vi "计算结果到报表.vi"(3 "计算参数":T1, 4 "试验模式":string, 5 "试验报表路径":path) -> ()   [LabVIEW 2013]
doc: "该函数将计算所得的参数写入到试验报表的文本文档里。"
uses:
  <vilib>/Utility/config.llb/Write Key (Double).vi
  <vilib>/Utility/config.llb/NI_LVConfig.lvlib
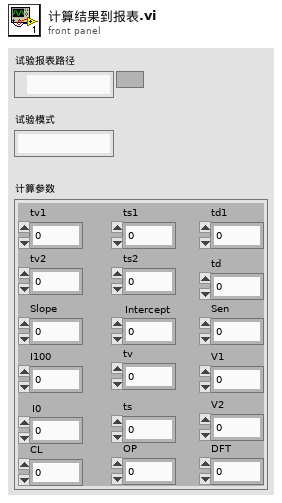
[diagram p1: front panel]
types:
  T1 = cluster{"tv1":dbl, "tv2":dbl, "tv":dbl, "ts1":dbl, "ts2":dbl, "ts":dbl, "td1":dbl, "td":dbl, "Slope":dbl, "Intercept":dbl, "I100":dbl, "I0":dbl, "Sen":dbl, "V1":dbl, "V2":dbl, "CL":dbl, "OP":dbl, "DFT":dbl}
  T2 = typedef "NI_LVConfig.lvlib/Config Data RefNum.ctl" = refnum<k1>
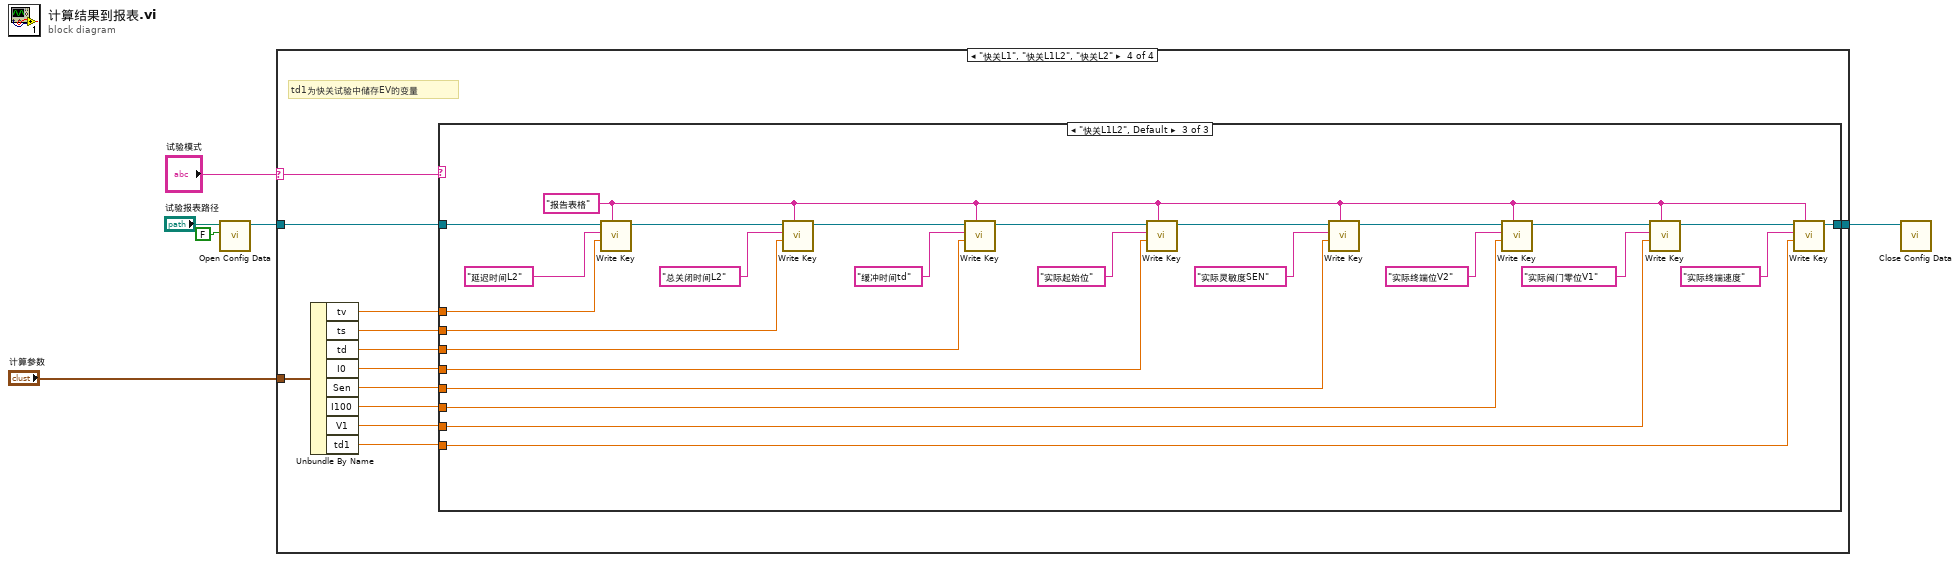
[diagram p0: block diagram]
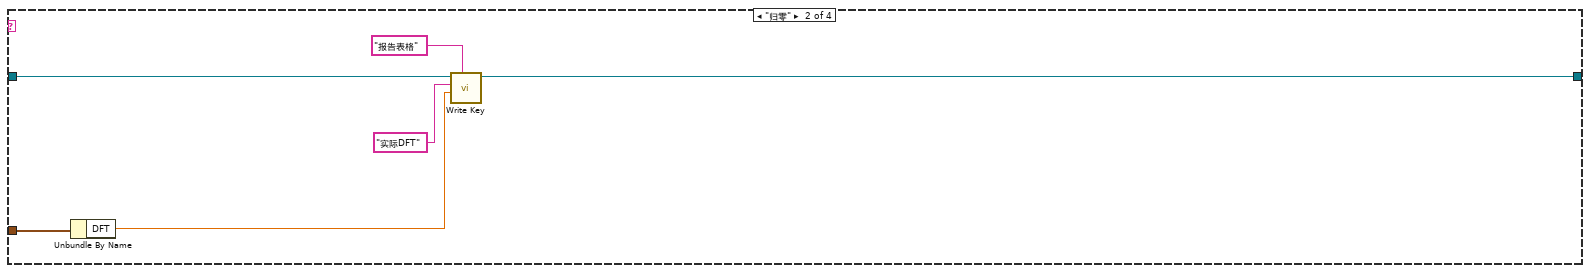
[diagram p3: hidden frame]
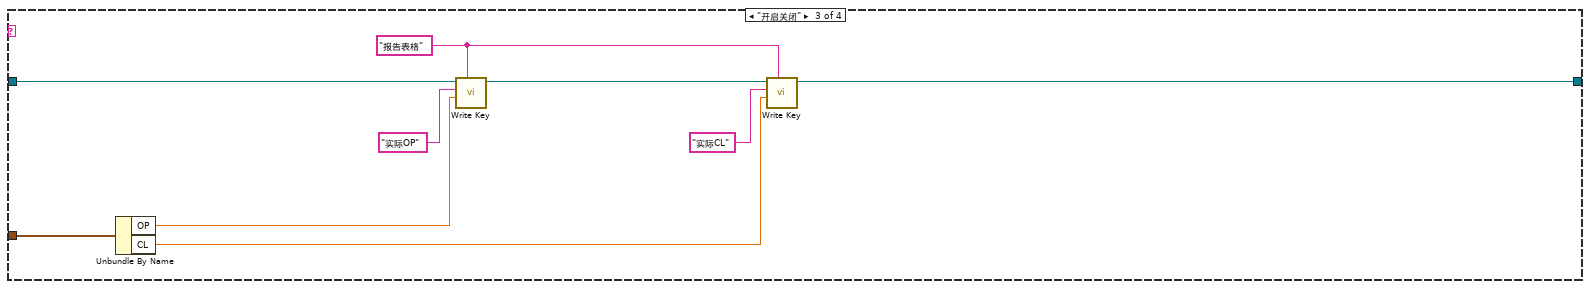
[diagram p4: hidden frame]
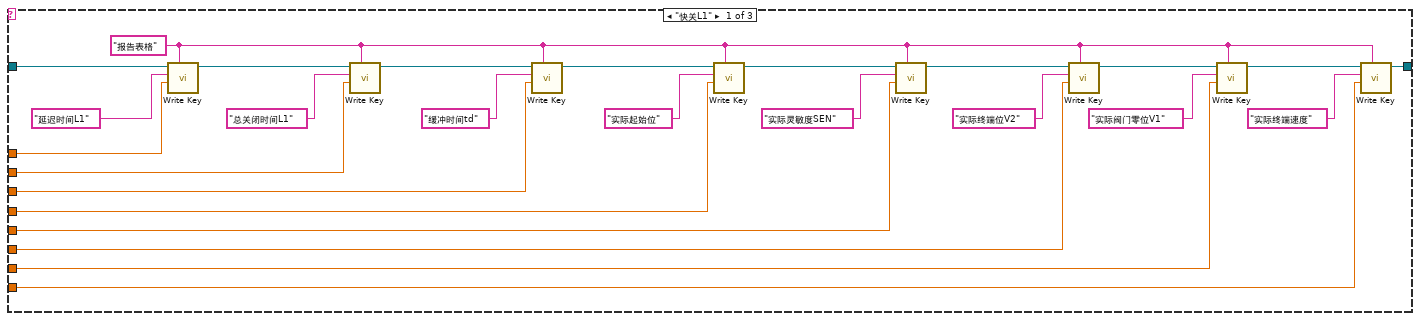
[diagram p5: hidden frame]
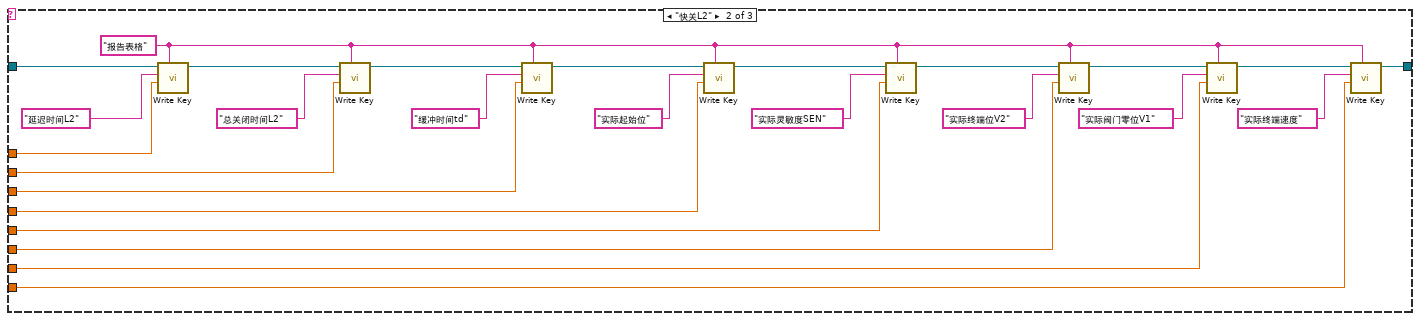
[diagram p6: hidden frame]
diagram:
  n1 = call <vilib>:"Open Config Data.vi"("create file if necessary (T)"=FALSE, "configuration file path"="试验报表路径") -> ("refnum"=w3:T2)  [unwired: 7 in, 2 out]
  n2 = case shown="\"快关L1\", \"快关L1L2\", \"快关L2\"" "试验模式" {
    selector: "试验模式" -> [_ _ _ w34]
    tunnel: "计算参数" -> [_ w13 w22 w33]
    tunnel: w3 -> [w7 w10 w15 w32]
    tunnel: [w7 w9 w14 w31] -> w2
    frame "步响应", Default {
    }
    frame "归零" {
      n3 = Unbundle By Name(w13) -> ("DFT"=w8:dbl)
      n4 = call-poly <vilib>:"Write Key.vi"("section"="报告表格", "value"=w8, "key"="实际DFT", "refnum"=w10) -> ("refnum out"=w9:T2)  [unwired: 5 in, 2 out]
    }
    frame "开启关闭" {
      w19 = "报告表格"
      n5 = Unbundle By Name(w22) -> ("OP"=w17:dbl, "CL"=w16:dbl)
      n6 = call-poly <vilib>:"Write Key.vi"("section"=w19, "value"=w17, "key"="实际OP", "refnum"=w15) -> ("refnum out"=w18:T2)  [unwired: 5 in, 2 out]
      n7 = call-poly <vilib>:"Write Key.vi"("section"=w19, "value"=w16, "key"="实际CL", "refnum"=w18) -> ("refnum out"=w14:T2)  [unwired: 5 in, 2 out]
    }
    frame "快关L1", "快关L1L2", "快关L2" {
      # "td1为快关试验中储存EV的变量"
      n8 = Unbundle By Name(w33) -> ("tv"=w30:dbl, "ts"=w29:dbl, "td"=w28:dbl, "I0"=w23:dbl, "Sen"=w24:dbl, "I100"=w25:dbl, "V1"=w26:dbl, "td1"=w27:dbl)
      n9 = case shown="\"快关L1L2\", Default" w34 {
        tunnel: w32 -> [w44 w86 w88]
        tunnel: [w43 w69 w87] -> w31
        tunnel: w30 -> [w35 w84 w89]
        tunnel: w29 -> [w36 w76 w90]
        tunnel: w28 -> [w37 w75 w91]
        tunnel: w23 -> [w38 w74 w92]
        tunnel: w24 -> [w39 w73 w93]
        tunnel: w25 -> [w40 w72 w94]
        tunnel: w26 -> [w41 w71 w95]
        tunnel: w27 -> [w42 w70 w96]
        frame "快关L1" {
          w45 = "报告表格"
          n10 = call-poly <vilib>:"Write Key.vi"("section"=w45, "value"=w35, "key"="延迟时间L1", "refnum"=w44) -> ("refnum out"=w52:T2)  [unwired: 5 in, 2 out]
          n11 = call-poly <vilib>:"Write Key.vi"("section"=w45, "value"=w36, "key"="总关闭时间L1", "refnum"=w52) -> ("refnum out"=w51:T2)  [unwired: 5 in, 2 out]
          n12 = call-poly <vilib>:"Write Key.vi"("section"=w45, "value"=w37, "key"="缓冲时间td", "refnum"=w51) -> ("refnum out"=w50:T2)  [unwired: 5 in, 2 out]
          n13 = call-poly <vilib>:"Write Key.vi"("section"=w45, "value"=w38, "key"="实际起始位", "refnum"=w50) -> ("refnum out"=w49:T2)  [unwired: 5 in, 2 out]
          n14 = call-poly <vilib>:"Write Key.vi"("section"=w45, "value"=w39, "key"="实际灵敏度SEN", "refnum"=w49) -> ("refnum out"=w48:T2)  [unwired: 5 in, 2 out]
          n15 = call-poly <vilib>:"Write Key.vi"("section"=w45, "value"=w40, "key"="实际终端位V2", "refnum"=w48) -> ("refnum out"=w47:T2)  [unwired: 5 in, 2 out]
          n16 = call-poly <vilib>:"Write Key.vi"("section"=w45, "value"=w41, "key"="实际阀门零位V1", "refnum"=w47) -> ("refnum out"=w46:T2)  [unwired: 5 in, 2 out]
          n17 = call-poly <vilib>:"Write Key.vi"("section"=w45, "value"=w42, "key"="实际终端速度", "refnum"=w46) -> ("refnum out"=w43:T2)  [unwired: 5 in, 2 out]
        }
        frame "快关L2" {
          w61 = "报告表格"
          n18 = call-poly <vilib>:"Write Key.vi"("section"=w61, "value"=w84, "key"="延迟时间L2", "refnum"=w86) -> ("refnum out"=w68:T2)  [unwired: 5 in, 2 out]
          n19 = call-poly <vilib>:"Write Key.vi"("section"=w61, "value"=w76, "key"="总关闭时间L2", "refnum"=w68) -> ("refnum out"=w67:T2)  [unwired: 5 in, 2 out]
          n20 = call-poly <vilib>:"Write Key.vi"("section"=w61, "value"=w75, "key"="缓冲时间td", "refnum"=w67) -> ("refnum out"=w66:T2)  [unwired: 5 in, 2 out]
          n21 = call-poly <vilib>:"Write Key.vi"("section"=w61, "value"=w74, "key"="实际起始位", "refnum"=w66) -> ("refnum out"=w65:T2)  [unwired: 5 in, 2 out]
          n22 = call-poly <vilib>:"Write Key.vi"("section"=w61, "value"=w73, "key"="实际灵敏度SEN", "refnum"=w65) -> ("refnum out"=w64:T2)  [unwired: 5 in, 2 out]
          n23 = call-poly <vilib>:"Write Key.vi"("section"=w61, "value"=w72, "key"="实际终端位V2", "refnum"=w64) -> ("refnum out"=w63:T2)  [unwired: 5 in, 2 out]
          n24 = call-poly <vilib>:"Write Key.vi"("section"=w61, "value"=w71, "key"="实际阀门零位V1", "refnum"=w63) -> ("refnum out"=w62:T2)  [unwired: 5 in, 2 out]
          n25 = call-poly <vilib>:"Write Key.vi"("section"=w61, "value"=w70, "key"="实际终端速度", "refnum"=w62) -> ("refnum out"=w69:T2)  [unwired: 5 in, 2 out]
        }
        frame "快关L1L2", Default {
          w97 = "报告表格"
          n26 = call-poly <vilib>:"Write Key.vi"("section"=w97, "value"=w89, "key"="延迟时间L2", "refnum"=w88) -> ("refnum out"=w104:T2)  [unwired: 5 in, 2 out]
          n27 = call-poly <vilib>:"Write Key.vi"("section"=w97, "value"=w90, "key"="总关闭时间L2", "refnum"=w104) -> ("refnum out"=w103:T2)  [unwired: 5 in, 2 out]
          n28 = call-poly <vilib>:"Write Key.vi"("section"=w97, "value"=w91, "key"="缓冲时间td", "refnum"=w103) -> ("refnum out"=w102:T2)  [unwired: 5 in, 2 out]
          n29 = call-poly <vilib>:"Write Key.vi"("section"=w97, "value"=w92, "key"="实际起始位", "refnum"=w102) -> ("refnum out"=w101:T2)  [unwired: 5 in, 2 out]
          n30 = call-poly <vilib>:"Write Key.vi"("section"=w97, "value"=w93, "key"="实际灵敏度SEN", "refnum"=w101) -> ("refnum out"=w100:T2)  [unwired: 5 in, 2 out]
          n31 = call-poly <vilib>:"Write Key.vi"("section"=w97, "value"=w94, "key"="实际终端位V2", "refnum"=w100) -> ("refnum out"=w99:T2)  [unwired: 5 in, 2 out]
          n32 = call-poly <vilib>:"Write Key.vi"("section"=w97, "value"=w95, "key"="实际阀门零位V1", "refnum"=w99) -> ("refnum out"=w98:T2)  [unwired: 5 in, 2 out]
          n33 = call-poly <vilib>:"Write Key.vi"("section"=w97, "value"=w96, "key"="实际终端速度", "refnum"=w98) -> ("refnum out"=w87:T2)  [unwired: 5 in, 2 out]
        }
      }
    }
  }
  n34 = call <vilib>:"Close Config Data.vi"("refnum"=w2) -> ()  [unwired: 9 in, 2 out]
